vi "deadzone.vi"(1 "threshold":dbl, 2 "in":dbl) -> (0 "out":dbl)   [LabVIEW 2009]
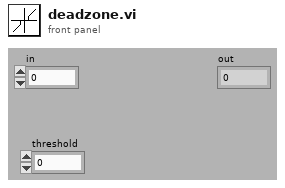
[diagram p1: front panel]
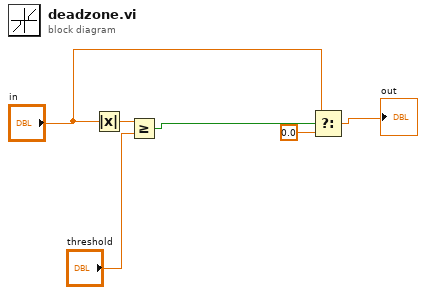
[diagram p0: block diagram]
diagram:
  n1 = Absolute Value(x="in") -> (abs(x)=w2:dbl)
  n2 = Greater Or Equal?(x=w2, y="threshold") -> (x >= y?=w5:bool)
  n3 = Select(t="in", s=w5, f=0.0) -> (s? t:f=→"out":dbl)
